vi "RQST Comm_Close All Connections.vi"(7 "Name":string, 8 "error in":errorcluster, 10 "ref in":T1, 11 "listener ID":refnum<k5>) -> (0 "error out":errorcluster)   [LabVIEW 2013, in "J1939 Addon Engine.lvlib"]
uses:
  Engine/J1939 Addon Engine.lvlib
  Types/RQST Comm Lookup Table_Ref.ctl
  STM/Connection Manager/stm_TCPConnectionMethod.ctl
  J1939 Addon Shared.lvlib
  <vilib>/NI Veristand/Custom Device Tools/Custom Device Utility Library/Custom Device Utility Library.lvlib
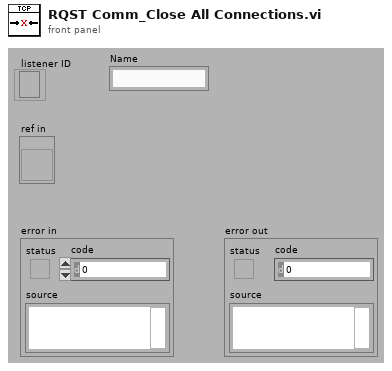
[diagram p1: front panel]
types:
  T1 = typedef "J1939 Addon Engine.lvlib/RQST Comm Lookup Table_Ref.ctl" = refnum<vi>
  T2 = typedef "J1939 Addon Shared.lvlib/stm_TCPConnectionMethod.ctl" = enum16{"Initialize", "Add Connection", "Set Properties", "Get Connection(s)", "Remove Connection", "Remove All Connections", "Get Connection Count"}
  T3 = typedef "J1939 Addon Shared.lvlib/stm_TCP Connection Info.ctl" = cluster{"connection ID":refnum<k5>, "Meta data":T4[]}
  T4 = typedef "J1939 Addon Shared.lvlib/stm_MetaDataElement.ctl" = string
  T5 = typedef "J1939 Addon Shared.lvlib/stm_TCPConnectionProperties.ctl" = cluster{"Name":string, "Address":string, "Custom":string}
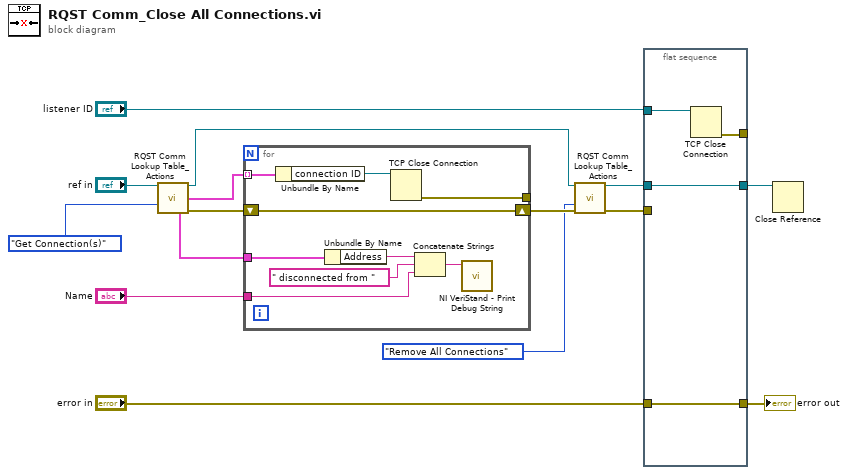
[diagram p0: block diagram]
diagram:
  n1 = call "RQST Comm Lookup Table_Actions.vi"("ref in"="ref in", "Method"=stm_TCPConnectionMethod."Get Connection(s)") -> ("reference out"=w3:T1, "All Connections"=w11:T3[], "Properties out"=w1:T5, "error out"=w10:errorcluster)  [unwired: 7 in, 3 out]
  n2 = for {
    tunnel: w11 -> [w16] mode=indexing
    shift-right: [w22] -> w9
    shift-left: w10 -> [w22]
    tunnel: [w23] -> _
    tunnel: "Name" -> [w18]
    tunnel: w1 -> [w17]
    n3 = Unbundle By Name(w16) -> ("connection ID"=w24:refnum<k5>)
    n4 = Unbundle By Name(w17) -> ("Address"=w19:string)
    n5 = TCP Close Connection(connection ID=w24) -> (error out=w23:errorcluster)  [unwired: 2 in, 1 out]
    n6 = Concatenate Strings(w19, " disconnected from " ("string"), w18) -> (w21:string)
    n7 = call <vilib>:"NI VeriStand - Print Debug String.vi"("Message"=w21) -> ()  [unwired: 10 in, 1 out]
  }
  n8 = call "RQST Comm Lookup Table_Actions.vi"("ref in"=w3, "Method"=stm_TCPConnectionMethod."Remove All Connections", "error in (no error)"=w9) -> ("reference out"=w5:T1, "error out"=w8:errorcluster)  [unwired: 6 in, 5 out]
  n9 = flat-sequence {
    tunnel: "listener ID" -> [w28]
    tunnel: [w27] -> w14
    tunnel: w8 -> [_]
    tunnel: "error in" -> [w27]
    tunnel: [w26] -> _
    tunnel: w5 -> [w25]
    tunnel: [w25] -> w4
    frame #0 {
      n10 = TCP Close Connection(connection ID=w28) -> (error out=w26:errorcluster)  [unwired: 2 in, 1 out]
    }
  }
  n11 = Close Reference(reference=w4) -> ()  [unwired: 1 in, 1 out]
  "error out" <- w14
